vi "NR DFT HOST and FPGA.vi"() -> ()   [LabVIEW 2014]
uses:
  <vilib>/FPGAPlugInAG/cRIO-9063/niLvFpga_Open_cRIO-9063.vi
  <vilib>/rvi/interface/common/dynamic/niFpgaDynamicAddResources.vi
  <vilib>/Utility/error.llb/Error Cluster From Error Code.vi
  <vilib>/rvi/errors/niLvFpgaAdjustHostInterfaceError.vi
  <vilib>/FPGAPlugInAG/Dynamic/niLvFpga_Close_Dynamic.vi
  <vilib>/rvi/interface/nirviOpenFPGA/nirviOpenFPGA.xnode
  FPGA Bitfiles/trailswithgps_FPGATarget_nonrecursiveakhi_iwueaVQ9jq4.lvbitx
  final programs/non recursive akhil.vi
  FPGA Bitfiles/trailswithgps_FPGATarget2_nonrecursiveakhi_uvvAtEd39bc.lvbitx
  final programs/non recursive akhil2.vi
  <vilib>/rvi/interface/nirviReadWriteControl/nirviReadWriteControl.xnode
  <vilib>/rvi/interface/nirviCloseFPGA/nirviCloseFPGA.xnode
  NiFpgaLv.dll
  <vilib>/rvi/interface/Simulation/niFpgaSimulationCallBeginRW.vi
panel:
  out "Apparent Power":dynamicdata(graph)
  out "Reactive Power":dynamicdata(graph)
  out "Real Power":dynamicdata(graph)
  out "Waveform Chart 4":dynamicdata(graph)
  out "x-y 3":fxp<+/-,50,26>
  out "x-y 2":fxp<+/-,49,25>
  out "x/y 4":fxp<+/-,48,24>
  out "x/y 3":fxp<+/-,48,24>
  out "Waveform Chart 3":dbl(graph)
  out "x-y":fxp<+/-,49,25>
  out "x/y 2":fxp<+/-,48,24>
  out "x/y":fxp<+/-,48,24>
  out "Load angle":dbl
  out "Load angle":dbl(graph)
  out "Apparent Power":dbl
  out "Power factor":dbl
  out "Real Power":dbl
  out "Reactive Power":dbl
  out "Apparent Power":dbl
  out "Power factor":dbl
  out "Real Power":dbl
  out "Reactive Power":dbl
  out "Frequency":dynamicdata(graph)
  out "ROCOF2":fxp<+/-,26,12>[](array[numeric])
  out "Frequency 2":fxp<+/-,50,19>[](array[numeric])
  out "Voltages at PMU 2":dynamicdata(graph)
  out "?":cluster{fxp<+,60,17>[]}[](array[cluster])
  out "?":cluster{fxp<+/-,22,10>[]}[](array[cluster])
  out "?":cluster{fxp<+,60,17>[]}[](array[cluster])
  out "?":cluster{fxp<+/-,22,10>[]}[](array[cluster])
  in  "polar attributes 9":T1={"maximum"=0.0, "minimum"=0.0, "clip to min"=FALSE, "log?(F)"=FALSE, "grid color"=6710886, "plot color"=65280, "fmt and prec"={"format"=enum."Decimal", "precision"=0}, "visible section"=8} {"minimum" format="%0.2f"; "maximum" format="%0.2f"}
  out "Voltage Phasors":picture
  in  "polar attributes 8":T1={"maximum"=0.0, "minimum"=0.0, "clip to min"=FALSE, "log?(F)"=FALSE, "grid color"=6710886, "plot color"=65280, "fmt and prec"={"format"=enum."Decimal", "precision"=0}, "visible section"=8} {"minimum" format="%0.2f"; "maximum" format="%0.2f"}
  out "Current Phasors":picture
  out "Magnitude 2":fxp<+,60,17>[](array[numeric])
  out "Theta 2":fxp<+/-,22,10>[](array[numeric])
  out "ROCOF":fxp<+/-,26,12>
  out "Altitude (m) 2":fxp<+/-,24,17>
  out "Longitude (°) 2":fxp<+/-,29,9>
  out "Latitude (°) 2":fxp<+/-,28,8>
  out "antenna status 2":T2(ring)
  out "PPS UTC Timestamp 2":timestamp format="%<%.9X\n%x>T"
  out "PPS TAI Timestamp 2":timestamp format="%<%.9X\n%x>T"
  out "PPS Timestamp (TAI ns) 2":u64
  out "phase current 2":fxp<+/-,17,17>
  out "current frequency 2":fxp<+/-,50,19>
  out "Frequency":fxp<+/-,50,19>
  out "UTC offset valid 2":bool
  out "UTC offset 2":i8
  out "Satellites Available 2":u8
  out "offset from time reference 2":i32
  out "FPGA Timekeeper locked 2":bool
  out "GPS status 2":T3(ring)
  out "phase voltage 2":fxp<+/-,17,17>
  out "LabVIEW time 2":timestamp
  out "Voltages at PMU 1":dynamicdata(graph)
  out "double precision float":dbl
  out "theta":dbl
  out "r":dbl
  out "element 2":fxp<+/-,25,11>
  out "element":fxp<+/-,25,11>
  out "subarray":fxp<+/-,25,11>[](array[numeric])
  out "sdft magnitude":fxp<+/-,25,11>[](array[numeric])
  out "sdft phase":fxp<+/-,25,11>[](array[numeric])
  out "sdft frequency":dbl
  out "a value":cdb
  out "?":cluster{fxp<+,60,17>[]}[](array[cluster])
  out "?":cluster{fxp<+/-,22,10>[]}[](array[cluster])
  out "?":cluster{fxp<+,60,17>[]}[](array[cluster])
  out "?":cluster{fxp<+/-,22,10>[]}[](array[cluster])
  in  "polar attributes 7":T1={"maximum"=0.0, "minimum"=0.0, "clip to min"=FALSE, "log?(F)"=FALSE, "grid color"=6710886, "plot color"=65280, "fmt and prec"={"format"=enum."Decimal", "precision"=0}, "visible section"=8} {"minimum" format="%0.2f"; "maximum" format="%0.2f"}
  out "Voltage Phasors":picture
  in  "polar attributes 6":T1={"maximum"=0.0, "minimum"=0.0, "clip to min"=FALSE, "log?(F)"=FALSE, "grid color"=6710886, "plot color"=65280, "fmt and prec"={"format"=enum."Decimal", "precision"=0}, "visible section"=8} {"minimum" format="%0.2f"; "maximum" format="%0.2f"}
  out "Current Phasors":picture
  out "Magnitude":fxp<+,60,17>[](array[numeric])
  out "Theta":fxp<+/-,22,10>[](array[numeric])
  out "ROCOF":fxp<+/-,26,12>[](array[numeric])
  out "ROCOF":fxp<+/-,26,12>
  out "Altitude (m)":fxp<+/-,24,17>
  out "Longitude (°)":fxp<+/-,29,9>
  out "Latitude (°)":fxp<+/-,28,8>
  out "Frequency":fxp<+/-,50,19>[](array[numeric])
  out "GPS TIMESTAMP":timestamp[](array[timestamp])
  out "antenna status":T2(ring)
  out "PPS UTC Timestamp":timestamp format="%<%.9X\n%x>T"
  out "PPS TAI Timestamp":timestamp format="%<%.9X\n%x>T"
  out "PPS Timestamp (TAI ns)":u64
  out "phase current":fxp<+/-,17,17>
  out "current frequency":fxp<+/-,50,19>
  out "Frequency":fxp<+/-,50,19>
  out "UTC offset valid":bool
  out "UTC offset":i8
  out "Satellites Available":u8
  out "offset from time reference":i32
  out "FPGA Timekeeper locked":bool
  out "GPS status":T3(ring)
  out "phase voltage":fxp<+/-,17,17>
  out "LabVIEW time":timestamp
  # "Phasor data concentrator"
  # "PHASOR DATA CONCENTRATOR (NON RECURSIVE ALGORITHM)"
  # "PHASOR MEASUREMENT UNIT 1"
  # "PHASOR MEASUREMENT UNIT 2"
  # "GPS SYNCHRONIZATION"
  # "Voltage Phasors"
  # "Voltage Phasors"
  # "R Phase"
  # "R Phase"
  # "Y Phase"
  # "Y Phase"
  # "B Phase"
  # "B Phase"
  # "Frequency and ROCOF"
  # "Frequency and ROCOF"
  # "Current Phasors"
  # "Current Phasors"
  # "R Phase"
  # "PMU 1"
  # "PMU 2"
  # "R Phase"
  # "Y Phase"
  # "Y Phase"
  # "B Phase"
  # "B Phase"
  # "PHASOR DATA CONCENTRATOR (NON RECURSIVE ALGORITHM)"
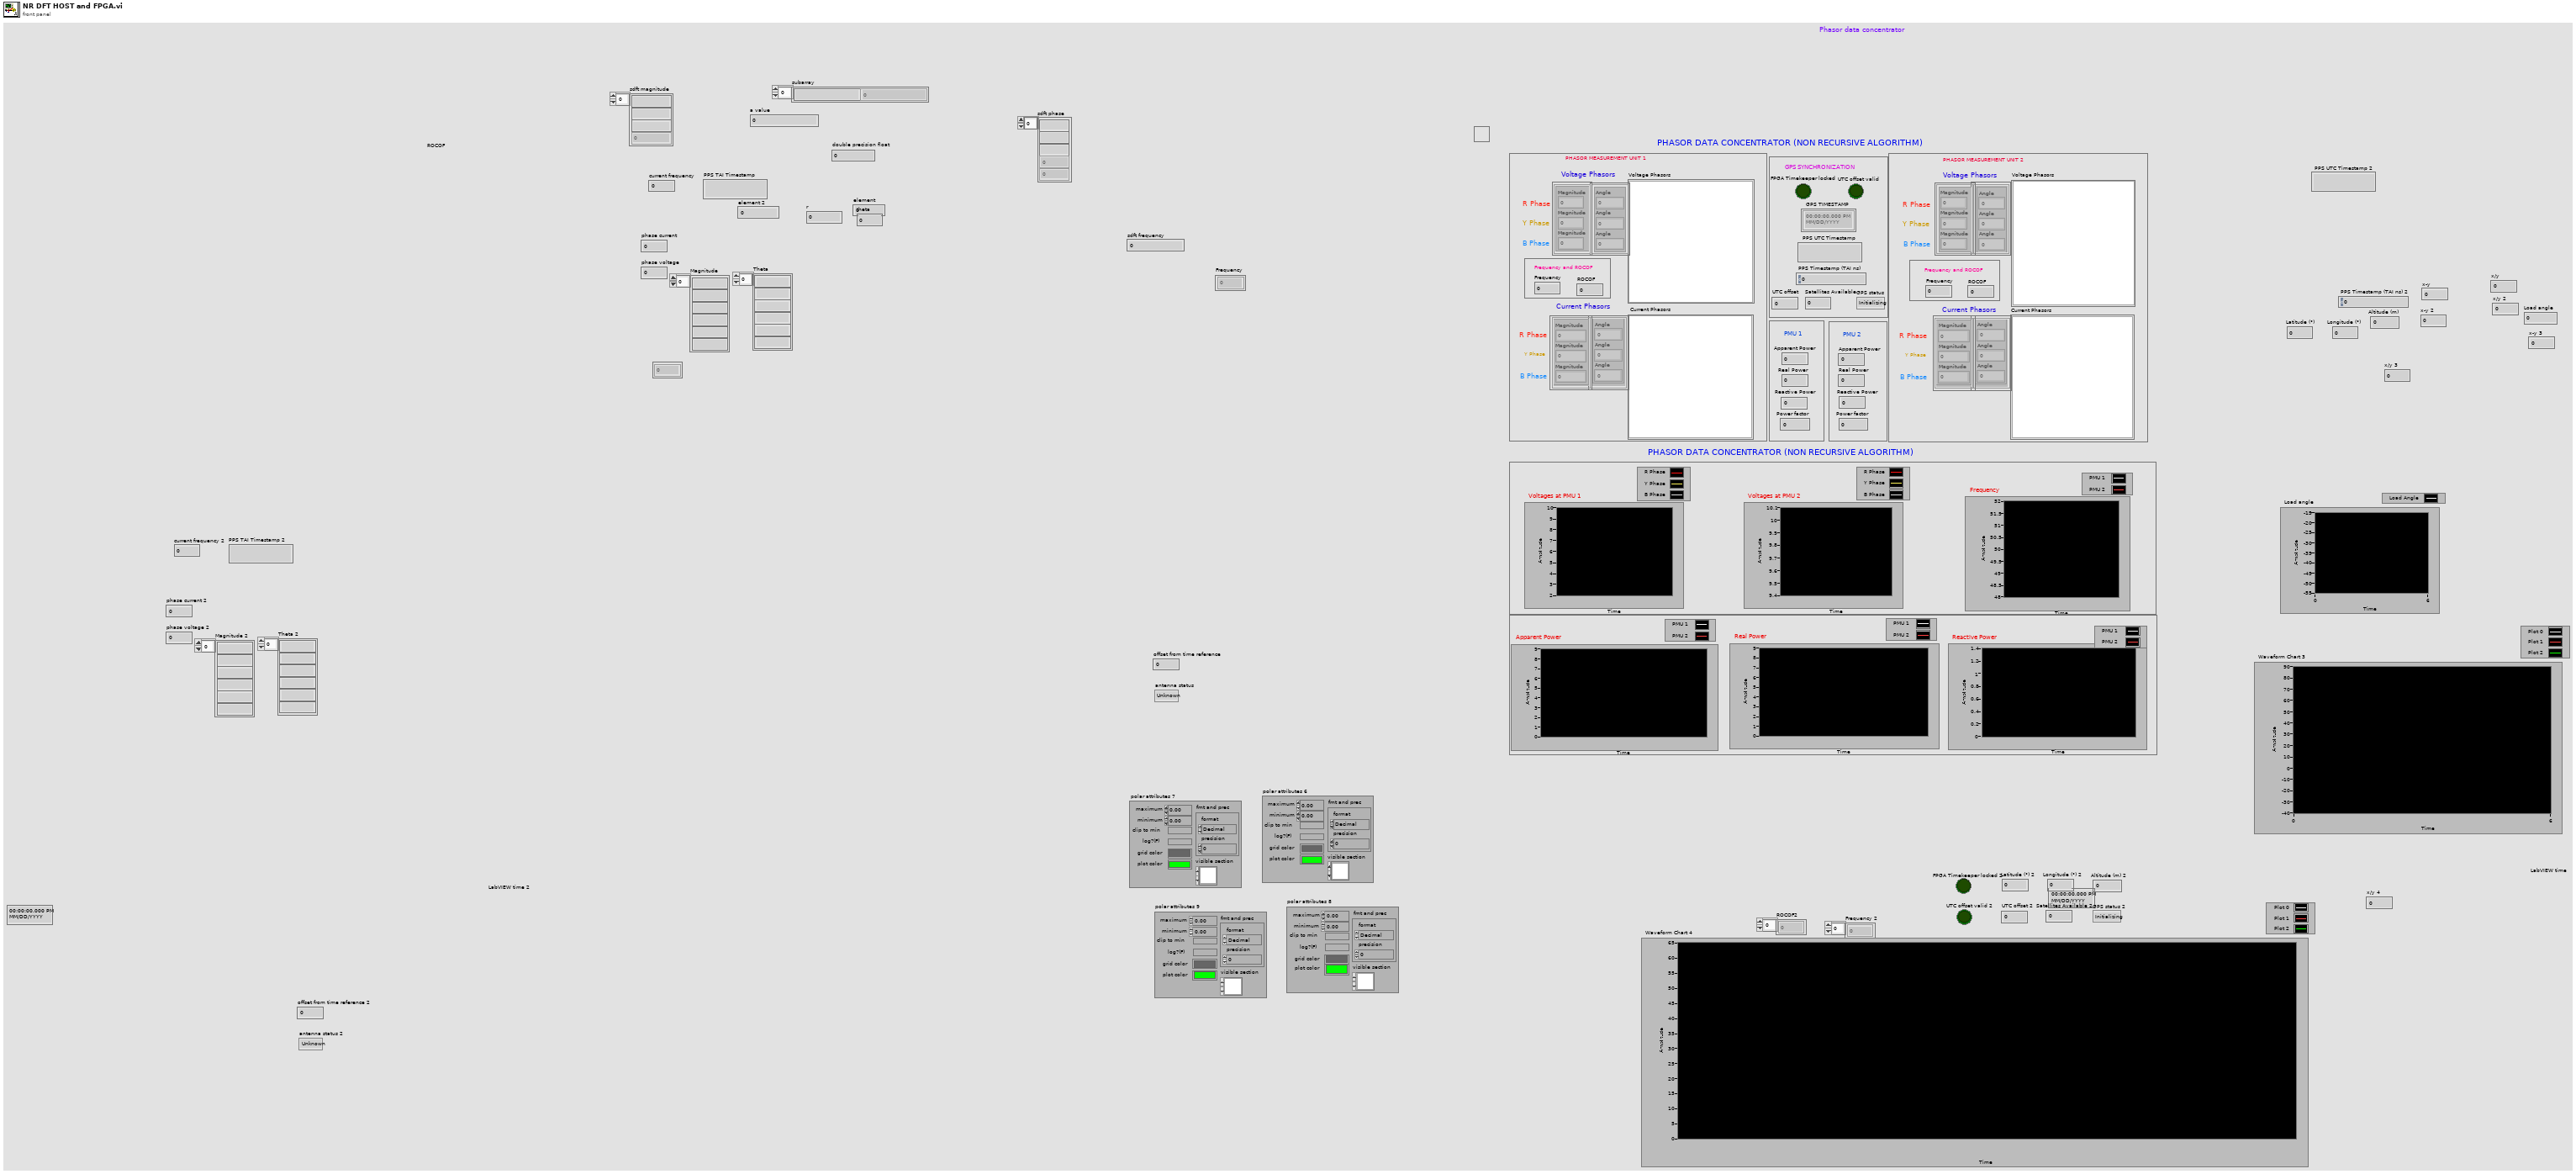
[diagram p1: front panel]
types:
  T1 = cluster{"maximum":dbl, "minimum":dbl, "clip to min":bool, "log?(F)":bool, "grid color":u32, "plot color":u32, "fmt and prec":cluster{"format":enum8{"Decimal", "Scientific", "Engineering", "Binary", "Octal", "Hex"}, "precision":u8}, "visible section":u16}
  T2 = enum8{"Unknown", "Normal", "Absent", "Overcurrent"}
  T3 = enum8{"Initializing", "Normal", "Unable to get fix"}
  T4 = cluster{"magnitude":fxp<+,60,17>, "element":fxp<+/-,61,18>}[]
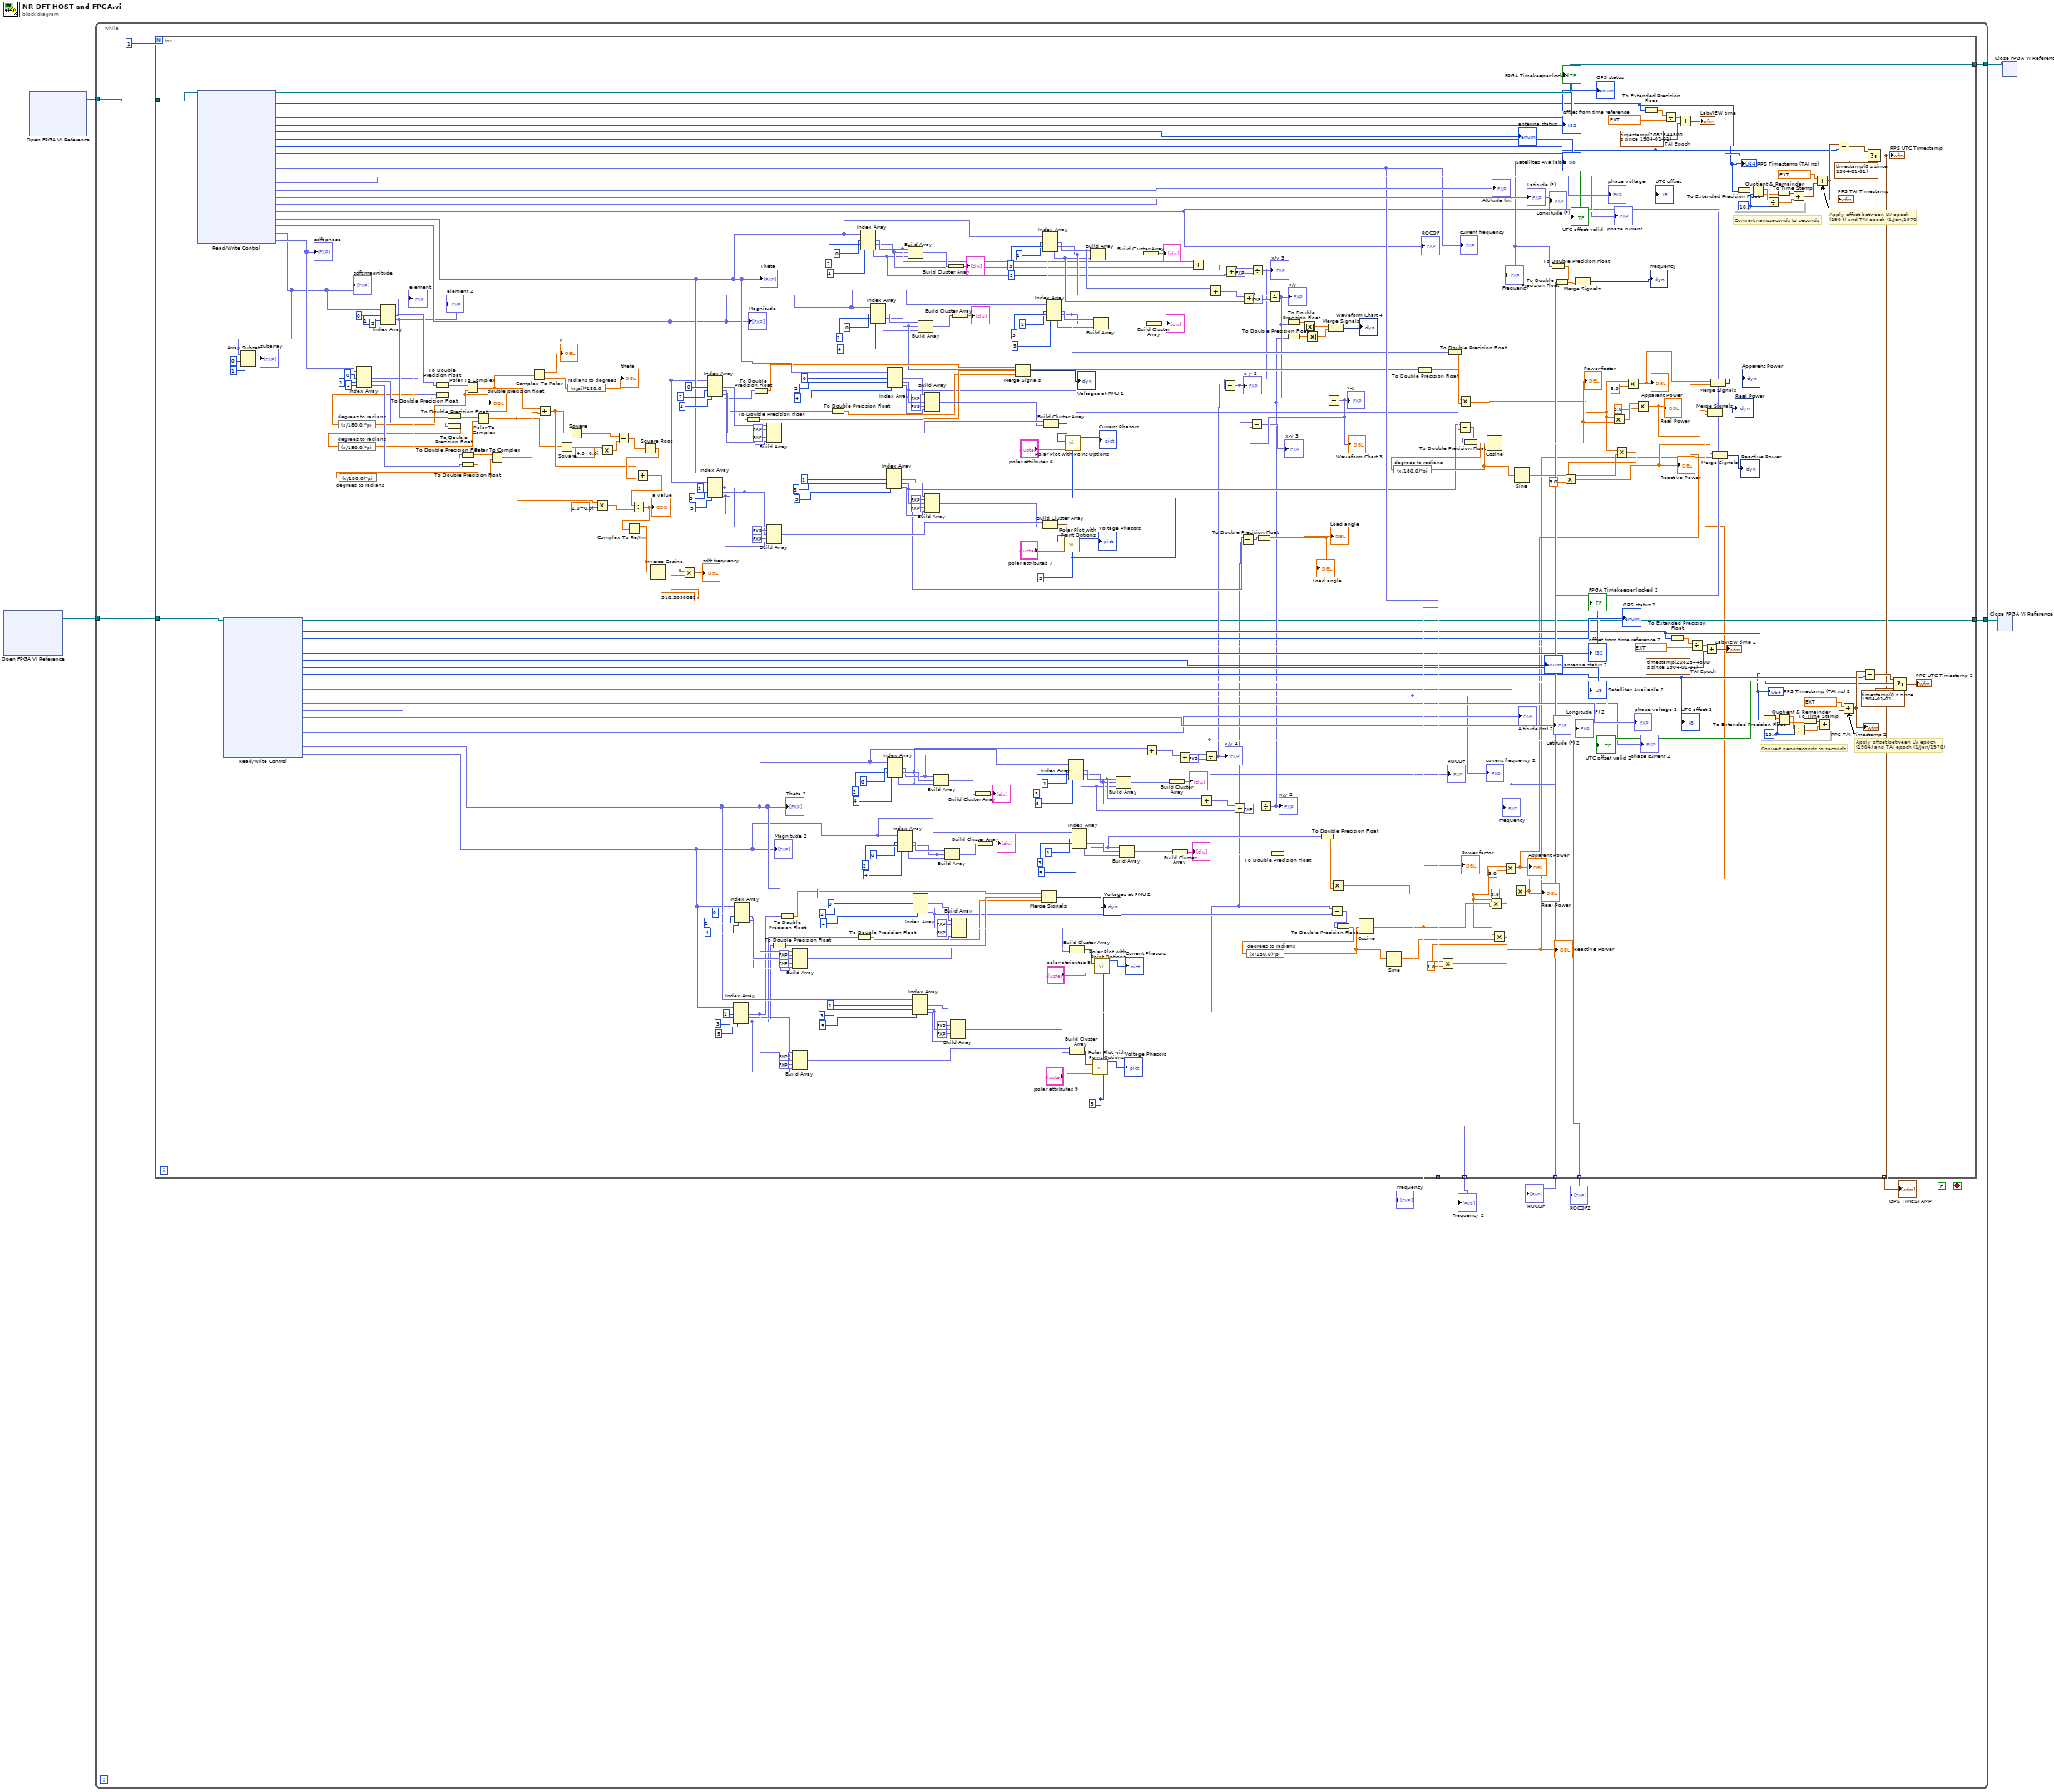
[diagram p0: block diagram]
diagram:
  n1 = xnode "Open FPGA VI Reference"() -> ("FPGA VI Reference Out"=w2:refnum<k20>)  [unwired: 2 in, 1 out]
  n2 = xnode "Open FPGA VI Reference"() -> ("FPGA VI Reference Out"=w3:refnum<k20>)  [unwired: 2 in, 1 out]
  n3 = while {
    tunnel: [w14] -> w4
    tunnel: w3 -> [w12]
    tunnel: w2 -> [w7]
    tunnel: [w5] -> w1
    stop <- FALSE stop-if-true
    n4 = for {
      N: 1 ("Numeric") -> [_]
      tunnel: w12 -> [w352]
      tunnel: [w351] -> w14
      tunnel: [w32] -> w15 mode=indexing
      tunnel: [w228] -> w11 mode=indexing
      tunnel: [w227] -> w10 mode=indexing
      tunnel: w7 -> [w128]
      tunnel: [w127] -> w9 mode=indexing
      tunnel: [w126] -> w8 mode=indexing
      tunnel: [w31] -> w5
      w70 = u16 5 ("Size 2")
      w275 = u16 5 ("Size")
      w206 = u32 1000000000
      w216 = timestamp(2082844800 s since 1904-01-01)  # TAI Epoch
      w344 = u32 1000000000
      w356 = timestamp(2082844800 s since 1904-01-01)  # TAI Epoch
      # "Apply offset between LV epoch (1904) and TAI epoch (1/Jan/1970)"
      # "Convert nanoseconds to seconds"
      # "Apply offset between LV epoch (1904) and TAI epoch (1/Jan/1970)"
      # "Convert nanoseconds to seconds"
      n5 = xnode "Read/Write Control"("FPGA VI Reference In"=w352) -> ("FPGA VI Reference Out"=w351:refnum<k20>, "FPGA Timekeeper time (ns)"=w332:u64, "GPS status"=→"GPS status":T3, "FPGA Timekeeper locked"=→"FPGA Timekeeper locked":bool, "offset from time reference"=→"offset from time reference":i32, "antenna status"=→"antenna status":T2, "satellites available"=→"Satellites Available":u8, "UTC offset"=w334:i8, "UTC offset valid"=w335:bool, "voltage frequency"=w109:fxp<+/-,50,19>, "current frequency"=w228:fxp<+/-,50,19>, "phase voltage"=→"phase voltage":fxp<+/-,26,12>, "phase current"=→"phase current":fxp<+/-,26,12>, "Latitude (°)"=→"Latitude (°)":fxp<+/-,28,8>, "Longitude (°)"=→"Longitude (°)":fxp<+/-,29,9>, "Altitude (m)"=→"Altitude (m)":fxp<+/-,24,17>, "rate of chage of frequency"=w227:fxp<+/-,26,12>, "theta"=w291:fxp<+/-,22,10>[], "r"=w284:fxp<+,60,17>[], "sdft magnitude"=w249:fxp<+/-,25,11>[], "sdft phase"=w269:fxp<+/-,25,11>[])  [unwired: 1 in, 1 out]
      "UTC offset" <- w334
      "UTC offset valid" <- w335
      "Frequency" <- w109
      "current frequency" <- w228
      "PPS Timestamp (TAI ns)" <- w332
      "ROCOF" <- w227
      "Theta" <- w291
      "Magnitude" <- w284
      "sdft phase" <- w269
      "sdft magnitude" <- w249
      n6 = xnode "Read/Write Control"("FPGA VI Reference In"=w128) -> ("FPGA VI Reference Out"=w31:refnum<k20>, "FPGA Timekeeper time (ns)"=w194:u64, "GPS status"=→"GPS status 2":T3, "FPGA Timekeeper locked"=→"FPGA Timekeeper locked 2":bool, "offset from time reference"=→"offset from time reference 2":i32, "antenna status"=→"antenna status 2":T2, "satellites available"=→"Satellites Available 2":u8, "UTC offset"=w196:i8, "UTC offset valid"=w197:bool, "voltage frequency"=w108:fxp<+/-,50,19>, "current frequency"=w127:fxp<+/-,50,19>, "phase voltage"=→"phase voltage 2":fxp<+/-,26,12>, "phase current"=→"phase current 2":fxp<+/-,26,12>, "Latitude (°)"=→"Latitude (°) 2":fxp<+/-,28,8>, "Longitude (°)"=→"Longitude (°) 2":fxp<+/-,29,9>, "Altitude (m)"=→"Altitude (m) 2":fxp<+/-,24,17>, "rate of chage of frequency"=w126:fxp<+/-,26,12>, "theta"=w155:fxp<+/-,22,10>[], "r"=w144:fxp<+,60,17>[])  [unwired: 1 in, 1 out]
      "UTC offset 2" <- w196
      "UTC offset valid 2" <- w197
      "Frequency" <- w108
      "current frequency 2" <- w127
      "PPS Timestamp (TAI ns) 2" <- w194
      "ROCOF" <- w126
      "Theta 2" <- w155
      "Magnitude 2" <- w144
      n7 = Array Subset(array=w249, index=0, length=1) -> (→"subarray":fxp<+/-,25,11>[])
      n8 = Index Array(array=w269, index #1=0 ("index"), index #2=1 ("index"), index #3=2 ("index")) -> (element #1=w238:fxp<+/-,25,11>, element #2=w242:fxp<+/-,25,11>, element #3=w241:fxp<+/-,25,11>)
      n9 = Index Array(array=w249, index #1=0 ("index"), index #2=1 ("index"), index #3=2 ("index")) -> (element #1=w245:fxp<+/-,25,11>, element #2=w244:fxp<+/-,25,11>, element #3=w243:fxp<+/-,25,11>)
      "element" <- w245
      "element 2" <- w244
      n10 = To Double Precision Float(number=w245) -> (double precision float=w267:dbl)
      n11 = To Double Precision Float(number=w238) -> (double precision float=w237:dbl)
      n12 = expression code="(x/180.0)*pi" "degrees to radians"(w237) -> (w236:dbl)
      "double precision float" <- w236
      n13 = To Double Precision Float(number=w244) -> (double precision float=w266:dbl)
      n14 = To Double Precision Float(number=w242) -> (double precision float=w235:dbl)
      n15 = expression code="(x/180.0)*pi" "degrees to radians"(w235) -> (w234:dbl)
      n16 = To Double Precision Float(number=w243) -> (double precision float=w265:dbl)
      n17 = To Double Precision Float(number=w241) -> (double precision float=w233:dbl)
      n18 = expression code="(x/180.0)*pi" "degrees to radians"(w233) -> (w225:dbl)
      n19 = Polar To Complex(1:w236, 2:w267) -> (0:w240:cdb)
      n20 = Polar To Complex(1:w234, 2:w266) -> (0:w256:cdb)
      n21 = Polar To Complex(1:w225, 2:w265) -> (0:w264:cdb)
      n22 = Complex To Polar(r * e^(i*theta)=w240) -> (r=→"r":dbl, theta=w232:dbl)
      n23 = Add(x=w240, y=w264) -> (x+y=w257:cdb)
      n24 = Square(x=w256) -> (x^2=w263:cdb)
      n25 = expression code="(x/pi)*180.0" "radians to degrees"(w232) -> (→"theta":dbl)
      n26 = Square(x=w257) -> (x^2=w260:cdb)
      n27 = Multiply(x=w256, y=cdb 2.0+0.0i) -> (x*y=w253:cdb)
      n28 = Multiply(x=w263, y=cdb 4.0+0.0i) -> (x*y=w261:cdb)
      n29 = Subtract(x=w260, y=w261) -> (x-y=w259:cdb)
      n30 = Square Root(x=w259) -> (sqrt(x)=w258:cdb)
      n31 = Add(x=w257, y=w258) -> (x+y=w254:cdb)
      n32 = Divide(x=w254, y=w253) -> (x/y=w252:cdb)
      "a value" <- w252
      n33 = Complex To Re/Im(x + iy=w252) -> (x=w251:dbl)  [unwired: 1 out]
      n34 = Inverse Cosine(1:w251) -> (0:w230:dbl)
      n35 = Multiply(x=w230, y=318.3098862) -> (x*y=→"sdft frequency":dbl)
      n36 = Index Array(array=w284, index #1=1 ("index"), index #2=3 ("index"), index #3=5 ("index")) -> (element #1=w21:fxp<+,60,17>, element #2=w20:fxp<+,60,17>, element #3=w19:fxp<+,60,17>)
      n37 = Index Array(array=w284, index #1=0 ("index"), index #2=2 ("index"), index #3=4 ("index")) -> (element #1=w223:fxp<+,60,17>, element #2=w226:fxp<+,60,17>, element #3=w221:fxp<+,60,17>)
      n38 = Index Array(array=w144, index #1=1 ("index"), index #2=3 ("index"), index #3=5 ("index")) -> (element #1=w18:fxp<+,60,17>, element #2=w17:fxp<+,60,17>, element #3=w16:fxp<+,60,17>)
      n39 = Index Array(array=w144, index #1=0 ("index"), index #2=2 ("index"), index #3=4 ("index")) -> (element #1=w133:fxp<+,60,17>, element #2=w135:fxp<+,60,17>, element #3=w131:fxp<+,60,17>)
      n40 = To Double Precision Float(number=w20) -> (double precision float=w224:dbl)
      n41 = To Double Precision Float(number=w21) -> (double precision float=w222:dbl)
      n42 = Build Array(w21, fxp<+,60,17> 0.0 ("element"), w20, fxp<+,60,17> 0.0 ("element"), w19) -> (w302:fxp<+,60,17>[])
      n43 = Build Array(w223, fxp<+,60,17> 0.0 ("element"), w226, fxp<+,60,17> 0.0 ("element"), w221) -> (w317:fxp<+,60,17>[])
      n44 = To Double Precision Float(number=w17) -> (double precision float=w134:dbl)
      n45 = To Double Precision Float(number=w18) -> (double precision float=w132:dbl)
      n46 = Build Array(w18, fxp<+,60,17> 0.0 ("element"), w17, fxp<+,60,17> 0.0 ("element"), w16) -> (w163:fxp<+,60,17>[])
      n47 = Build Array(w133, fxp<+,60,17> 0.0 ("element"), w135, fxp<+,60,17> 0.0 ("element"), w131) -> (w177:fxp<+,60,17>[])
      n48 = To Double Precision Float(number=w19) -> (double precision float=w220:dbl)
      n49 = To Double Precision Float(number=w16) -> (double precision float=w130:dbl)
      n50 = Index Array(array=w291, index #1=0 ("index"), index #2=2 ("index"), index #3=4 ("index")) -> (element #1=w54:fxp<+/-,22,10>, element #2=w53:fxp<+/-,22,10>, element #3=w52:fxp<+/-,22,10>)
      n51 = Index Array(array=w284, index #1=0 ("index"), index #2=2 ("index"), index #3=4 ("index")) -> (element #1=w123:fxp<+,60,17>, element #2=w115:fxp<+,60,17>, element #3=w110:fxp<+,60,17>)
      n52 = Index Array(array=w291, index #1=1 ("index"), index #2=3 ("index"), index #3=5 ("index")) -> (element #1=w125:fxp<+/-,22,10>, element #2=w81:fxp<+/-,22,10>, element #3=w112:fxp<+/-,22,10>)
      n53 = Index Array(array=w291, index #1=0 ("index"), index #2=2 ("index"), index #3=4 ("index")) -> (element #1=w124:fxp<+/-,22,10>, element #2=w116:fxp<+/-,22,10>, element #3=w113:fxp<+/-,22,10>)
      n54 = Index Array(array=w155, index #1=0 ("index"), index #2=2 ("index"), index #3=4 ("index")) -> (element #1=w47:fxp<+/-,22,10>, element #2=w48:fxp<+/-,22,10>, element #3=w46:fxp<+/-,22,10>)
      n55 = Index Array(array=w144, index #1=0 ("index"), index #2=2 ("index"), index #3=4 ("index")) -> (element #1=w148:fxp<+,60,17>, element #2=w91:fxp<+,60,17>, element #3=w149:fxp<+,60,17>)
      n56 = Build Array(w54, w53, w52) -> (w283:fxp<+/-,22,10>[])
      n57 = Index Array(array=w155, index #1=1 ("index"), index #2=3 ("index"), index #3=5 ("index")) -> (element #1=w165:fxp<+/-,22,10>, element #2=w80:fxp<+/-,22,10>, element #3=w164:fxp<+/-,22,10>)
      n58 = Index Array(array=w155, index #1=0 ("index"), index #2=2 ("index"), index #3=4 ("index")) -> (element #1=w179:fxp<+/-,22,10>, element #2=w90:fxp<+/-,22,10>, element #3=w178:fxp<+/-,22,10>)
      n59 = Build Array(w123, w115, w110) -> (w282:fxp<+,60,17>[])
      n60 = Build Array(w125, fxp<+,60,17> 0.0 ("element"), w81, fxp<+,60,17> 0.0 ("element"), w112) -> (w301:fxp<+/-,61,18>[])
      n61 = Build Array(w124, fxp<+,60,17> 0.0 ("element"), w116, fxp<+,60,17> 0.0 ("element"), w113) -> (w316:fxp<+/-,61,18>[])
      n62 = Build Array(w47, w48, w46) -> (w143:fxp<+/-,22,10>[])
      n63 = Build Array(w148, w91, w149) -> (w142:fxp<+,60,17>[])
      n64 = Build Cluster Array(w283) -> (→"?":cluster{fxp<+/-,22,10>[]}[])
      n65 = Build Array(w165, fxp<+,60,17> 0.0 ("element"), w80, fxp<+,60,17> 0.0 ("element"), w164) -> (w162:fxp<+/-,61,18>[])
      n66 = Build Array(w179, fxp<+,60,17> 0.0 ("element"), w90, fxp<+,60,17> 0.0 ("element"), w178) -> (w176:fxp<+/-,61,18>[])
      n67 = Build Cluster Array(w282) -> (→"?":cluster{fxp<+,60,17>[]}[])
      n68 = Build Cluster Array(w143) -> (→"?":cluster{fxp<+/-,22,10>[]}[])
      n69 = Build Cluster Array(w142) -> (→"?":cluster{fxp<+,60,17>[]}[])
      n70 = Merge Signals(w222, w224, w220) -> (→"Voltages at PMU 1":dynamicdata)
      n71 = Merge Signals(w132, w134, w130) -> (→"Voltages at PMU 2":dynamicdata)
      n72 = Index Array(array=w291, index #1=1 ("index"), index #2=3 ("index"), index #3=5 ("index")) -> (element #1=w69:fxp<+/-,22,10>, element #2=w68:fxp<+/-,22,10>, element #3=w66:fxp<+/-,22,10>)
      n73 = Build Cluster Array(w302, w301) -> (w299:T4)
      n74 = Build Cluster Array(w317, w316) -> (w314:T4)
      n75 = Index Array(array=w284, index #1=1 ("index"), index #2=3 ("index"), index #3=5 ("index")) -> (element #1=w122:fxp<+,60,17>, element #2=w114:fxp<+,60,17>, element #3=w111:fxp<+,60,17>)
      n76 = call <vilib>:"Polar Plot with Point Options.vi"("data array [mag, phase (deg)]"=w299, "polar attributes"="polar attributes 7", "Size"=w275) -> ("new picture"=→"Voltage Phasors":picture)  [unwired: 12 in]
      n77 = call <vilib>:"Polar Plot with Point Options.vi"("data array [mag, phase (deg)]"=w314, "polar attributes"="polar attributes 6", "Size"=w275) -> ("new picture"=→"Current Phasors":picture)  [unwired: 12 in]
      n78 = Index Array(array=w155, index #1=1 ("index"), index #2=3 ("index"), index #3=5 ("index")) -> (element #1=w60:fxp<+/-,22,10>, element #2=w59:fxp<+/-,22,10>, element #3=w58:fxp<+/-,22,10>)
      n79 = Build Cluster Array(w163, w162) -> (w76:T4)
      n80 = Build Cluster Array(w177, w176) -> (w73:T4)
      n81 = Index Array(array=w144, index #1=1 ("index"), index #2=3 ("index"), index #3=5 ("index")) -> (element #1=w92:fxp<+,60,17>, element #2=w153:fxp<+,60,17>, element #3=w154:fxp<+,60,17>)
      n82 = Build Array(w69, w68, w66) -> (w279:fxp<+/-,22,10>[])
      n83 = call <vilib>:"Polar Plot with Point Options.vi"("data array [mag, phase (deg)]"=w76, "polar attributes"="polar attributes 9", "Size"=w70) -> ("new picture"=→"Voltage Phasors":picture)  [unwired: 12 in]
      n84 = Build Array(w122, w114, w111) -> (w278:fxp<+,60,17>[])
      n85 = call <vilib>:"Polar Plot with Point Options.vi"("data array [mag, phase (deg)]"=w73, "polar attributes"="polar attributes 8", "Size"=w70) -> ("new picture"=→"Current Phasors":picture)  [unwired: 12 in]
      n86 = Build Array(w60, w59, w58) -> (w139:fxp<+/-,22,10>[])
      n87 = Build Array(w92, w153, w154) -> (w138:fxp<+,60,17>[])
      n88 = Build Cluster Array(w279) -> (→"?":cluster{fxp<+/-,22,10>[]}[])
      n89 = Add(x=w48, y=w47) -> (x+y=w51:fxp<+/-,23,11>)
      n90 = Build Cluster Array(w278) -> (→"?":cluster{fxp<+,60,17>[]}[])
      n91 = Build Cluster Array(w139) -> (→"?":cluster{fxp<+/-,22,10>[]}[])
      n92 = Build Cluster Array(w138) -> (→"?":cluster{fxp<+,60,17>[]}[])
      n93 = Add(x=w51, y=w46) -> (x+y=w50:fxp<+/-,24,12>)
      n94 = Add(x=w54, y=w53) -> (x+y=w57:fxp<+/-,23,11>)
      n95 = Add(x=w60, y=w59) -> (x+y=w63:fxp<+/-,23,11>)
      n96 = Divide(x=w50, y=fxp<+/-,24,12> 3.0) -> (x/y=w44:fxp<+/-,48,24>)
      "x/y 4" <- w44
      n97 = Add(x=w69, y=w68) -> (x+y=w67:fxp<+/-,23,11>)
      n98 = Add(x=w57, y=w52) -> (x+y=w56:fxp<+/-,24,12>)
      n99 = Add(x=w63, y=w58) -> (x+y=w62:fxp<+/-,24,12>)
      n100 = Subtract(x=w81, y=w80) -> (x-y=w79:fxp<+/-,23,11>)
      n101 = Add(x=w67, y=w66) -> (x+y=w65:fxp<+/-,24,12>)
      n102 = Divide(x=w56, y=fxp<+/-,24,12> 3.0) -> (x/y=w45:fxp<+/-,48,24>)
      "x/y 3" <- w45
      n103 = Subtract(x=w44, y=w45) -> (x-y=w43:fxp<+/-,49,25>)
      "x-y 2" <- w43
      n104 = To Double Precision Float(number=w79) -> (double precision float=→"Load angle" →"Load angle":dbl)
      n105 = Divide(x=w62, y=fxp<+/-,24,12> 3.0) -> (x/y=w39:fxp<+/-,48,24>)
      "x/y 2" <- w39
      n106 = Divide(x=w65, y=fxp<+/-,24,12> 3.0) -> (x/y=w40:fxp<+/-,48,24>)
      "x/y" <- w40
      n107 = To Double Precision Float(number=w91) -> (double precision float=w95:dbl)
      n108 = To Double Precision Float(number=w40) -> (double precision float=w38:dbl)
      n109 = To Double Precision Float(number=w39) -> (double precision float=w37:dbl)
      n110 = Absolute Value(x=w38) -> (abs(x)=w35:dbl)
      n111 = Absolute Value(x=w37) -> (abs(x)=w34:dbl)
      n112 = To Double Precision Float(number=w92) -> (double precision float=w96:dbl)
      n113 = Subtract(x=w40, y=w39) -> (x-y=w42:fxp<+/-,49,25>)
      "x-y" <- w42
      "Waveform Chart 3" <- w42
      n114 = Subtract(x=w43, y=w42) -> (x-y=→"x-y 3":fxp<+/-,50,26>)
      n115 = Merge Signals(w35, w34) -> (→"Waveform Chart 4":dynamicdata)
      n116 = Subtract(x=w80, y=w90) -> (x-y=w97:fxp<+/-,23,11>)
      n117 = Multiply(x=w95, y=w96) -> (x*y=w82:dbl)
      n118 = To Double Precision Float(number=w97) -> (double precision float=w93:dbl)
      n119 = expression code="(x/180.0)*pi" "degrees to radians"(w93) -> (w94:dbl)
      n120 = Cosine(x=w94) -> (cos(x)=w83:dbl)
      "Power factor" <- w83
      n121 = Sine(x=w94) -> (sin(x)=w85:dbl)
      n122 = To Double Precision Float(number=w115) -> (double precision float=w118:dbl)
      n123 = To Double Precision Float(number=w114) -> (double precision float=w119:dbl)
      n124 = Subtract(x=w81, y=w116) -> (x-y=w121:fxp<+/-,23,11>)
      n125 = Multiply(x=w118, y=w119) -> (x*y=w99:dbl)
      n126 = To Double Precision Float(number=w121) -> (double precision float=w117:dbl)
      n127 = expression code="(x/180.0)*pi" "degrees to radians"(w117) -> (w105:dbl)
      n128 = Cosine(x=w105) -> (cos(x)=w120:dbl)
      "Power factor" <- w120
      n129 = Multiply(x=w82, y=w83) -> (x*y=w89:dbl)
      n130 = Multiply(x=w82, y=w85) -> (x*y=w84:dbl)
      n131 = Multiply(x=w84, y=3.0) -> (x*y=w27:dbl)
      "Reactive Power" <- w27
      n132 = Multiply(x=w82, y=3.0) -> (x*y=w23:dbl)
      "Apparent Power" <- w23
      n133 = Multiply(x=w89, y=3.0) -> (x*y=w29:dbl)
      "Real Power" <- w29
      n134 = Sine(x=w105) -> (sin(x)=w104:dbl)
      n135 = To Double Precision Float(number=w109) -> (double precision float=w78:dbl)
      n136 = To Double Precision Float(number=w108) -> (double precision float=w107:dbl)
      n137 = Merge Signals(w78, w107) -> (→"Frequency":dynamicdata)
      n138 = Multiply(x=w99, y=w120) -> (x*y=w101:dbl)
      n139 = Multiply(x=w99, y=w104) -> (x*y=w103:dbl)
      n140 = Multiply(x=w103, y=3.0) -> (x*y=w28:dbl)
      "Reactive Power" <- w28
      n141 = Multiply(x=w99, y=3.0) -> (x*y=w24:dbl)
      "Apparent Power" <- w24
      n142 = Multiply(x=w101, y=3.0) -> (x*y=w30:dbl)
      "Real Power" <- w30
      n143 = To Extended Precision Float(1:w332) -> (0:w354:ext)
      n144 = Divide(x=w354, y=ext 1000000000.0) -> (x/y=w357:ext)
      n145 = To Extended Precision Float(1:w194) -> (0:w214:ext)
      n146 = Add(x=w357, y=w356) -> (x+y=→"LabVIEW time":timestamp)
      n147 = Divide(x=w214, y=ext 1000000000.0) -> (x/y=w217:ext)
      n148 = Add(x=w217, y=w216) -> (x+y=→"LabVIEW time 2":timestamp)
      n149 = Merge Signals(w30, w29) -> (→"Real Power":dynamicdata)
      n150 = Merge Signals(w24, w23) -> (→"Apparent Power":dynamicdata)
      n151 = Merge Signals(w28, w27) -> (→"Reactive Power":dynamicdata)
      n152 = To Extended Precision Float(1:w332) -> (0:w346:ext)
      n153 = Quotient & Remainder(x=w346, y=w344) -> (x-y*floor(x/y)=w345:ext, floor(x/y)=w343:ext)
      n154 = To Extended Precision Float(1:w194) -> (0:w208:ext)
      n155 = Divide(x=w345, y=w344) -> (x/y=w341:ext)
      n156 = To Time Stamp(1:w343) -> (0:w342:timestamp)
      n157 = Quotient & Remainder(x=w208, y=w206) -> (x-y*floor(x/y)=w207:ext, floor(x/y)=w205:ext)
      n158 = Add(x=w342, y=w341) -> (x+y=w340:timestamp)
      n159 = Divide(x=w207, y=w206) -> (x/y=w203:ext)
      n160 = To Time Stamp(1:w205) -> (0:w204:timestamp)
      n161 = Add(x=ext 2082844800.0, y=w340) -> (x+y=w338:timestamp)
      "PPS TAI Timestamp" <- w338
      n162 = Add(x=w204, y=w203) -> (x+y=w202:timestamp)
      n163 = Subtract(x=w338, y=w334) -> (x-y=w337:timestamp)
      n164 = Add(x=ext 2082844800.0, y=w202) -> (x+y=w200:timestamp)
      "PPS TAI Timestamp 2" <- w200
      n165 = Subtract(x=w200, y=w196) -> (x-y=w199:timestamp)
      n166 = Select(t=w337, s=w335, f=timestamp(0 s since 1904-01-01)) -> (s? t:f=w32:timestamp)
      "PPS UTC Timestamp" <- w32
      n167 = Select(t=w199, s=w197, f=timestamp(0 s since 1904-01-01)) -> (s? t:f=→"PPS UTC Timestamp 2":timestamp)
    }
    "GPS TIMESTAMP" <- w15
    "Frequency" <- w11
    "ROCOF" <- w10
    "Frequency 2" <- w9
    "ROCOF2" <- w8
  }
  n168 = xnode "Close FPGA VI Reference"("FPGA VI Reference In"=w1) -> ()  [unwired: 1 in, 1 out]
  n169 = xnode "Close FPGA VI Reference"("FPGA VI Reference In"=w4) -> ()  [unwired: 1 in, 1 out]
